vi "Attenuator_Test.vi"() -> ()   [LabVIEW 2018]
panel:
  in  "角度":i32=3000
  in  "轴":i32=2
  out "通信成功？":bool
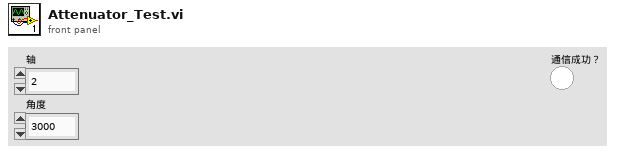
[diagram p1: front panel]
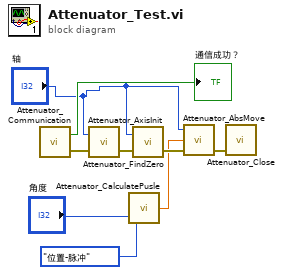
[diagram p0: block diagram]
diagram:
  n1 = call "Attenuator_Communication.vi"() -> ("错误输出"=w9:errorcluster, "通信成功？"=→"通信成功？":bool)  [unwired: 2 in]
  n2 = call "Attenuator_AxisInit.vi"("error in (no error)"=w9, "Axis"="轴") -> ("error out"=w6:errorcluster)  [unwired: 1 in]
  n3 = call "Attenuator_CalculatePusle.vi"("计算状态"=enum32{"位置-脉冲", "脉冲-位置"}."位置-脉冲", "数据"="角度") -> ("dataout"=w1:dbl)  [unwired: 2 in]
  n4 = call "Attenuator_FindZero.vi"("error in (no error)"=w6, "Axis"="轴") -> ("error out"=w5:errorcluster)  [unwired: 1 in]
  n5 = call "Attenuator_AbsMove.vi"("error in (no error)"=w5, "Deg"=w1, "Axis"="轴") -> ("error out"=w7:errorcluster)  [unwired: 2 in]
  n6 = call "Attenuator_Close.vi"("error in (no error)"=w7) -> ()  [unwired: 4 in, 1 out]
